vi "Excel_Quit.vi"(0 "Excel._Application in":refnum<k7>, 5 "Excel._Workbook in":refnum<k7>, 7 "save changes?":bool, 11 "error in":errorcluster, 12 "Close Application":bool, 13 "Close Report":bool) -> (4 "Excel._Application out":refnum<k7>, 6 "Excel._Workbook out":refnum<k7>, 15 "error out":errorcluster)   [LabVIEW 2020, in "NI_ReportGenerationToolkit.lvlib"]
uses:
  <vilib>/addons/_office/NI_ReportGenerationToolkit.lvlib
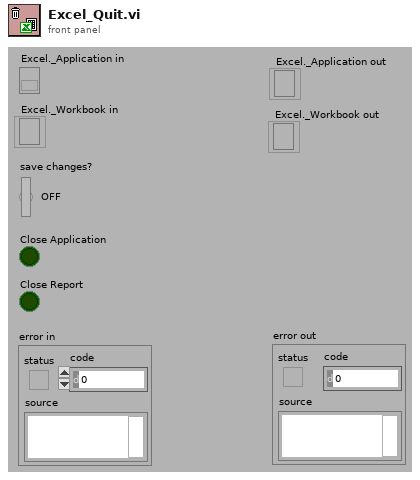
[diagram p1: front panel]
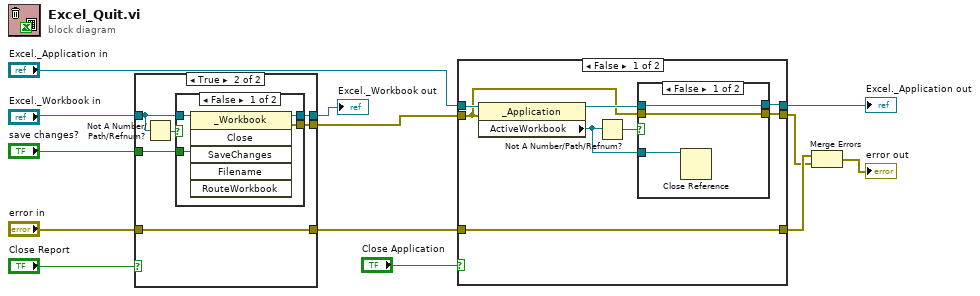
[diagram p0: block diagram]
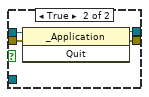
[diagram p2: hidden frame]
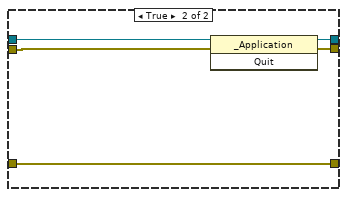
[diagram p3: hidden frame]
diagram:
  n1 = case shown="True" "Close Report" {
    tunnel: "save changes?" -> [_ w21]
    tunnel: [w14 w20] -> w4
    tunnel: "error in" -> [w14 w20]
    tunnel: "Excel._Workbook in" -> [w15 w17]
    tunnel: [w15 w19] -> w6
    tunnel: [_ w18] -> w3
    frame False {
    }
    frame True {
      n2 = Not A Number/Path/Refnum?(number/path/refnum=w17) -> (NaN/Path/Refnum?=w16:bool)
      n3 = case shown="False" w16 {
        tunnel: w21 -> [w25 _]
        tunnel: w17 -> [w24 w26]
        tunnel: [w23 w26] -> w19
        tunnel: [w22 _] -> w18
        frame False {
          n4 = invoke class="_Workbook" method="Close"(reference=w24, "SaveChanges"=w25) -> (reference out=w23:refnum<k7>, error out=w22:errorcluster)  [unwired: 4 in, 4 out]
        }
        frame True {
        }
      }
    }
  }
  "Excel._Workbook out" <- w6
  n5 = case shown="False" "Close Application" {
    tunnel: [w33 w46] -> w12
    tunnel: [w32 w45] -> w1
    tunnel: w4 -> [w34 w44]
    tunnel: [w34 w44] -> w2
    tunnel: "Excel._Application in" -> [w31 w43]
    tunnel: w3 -> [w28 w42]
    frame False {
      n6 = property class="_Application"(reference=w31, error in=w28) -> (reference out=w30:refnum<k7>, "ActiveWorkbook"=w27:refnum<k7>)  [unwired: 1 out]
      n7 = Not A Number/Path/Refnum?(number/path/refnum=w27) -> (NaN/Path/Refnum?=w29:bool)
      n8 = case shown="False" w29 {
        tunnel: [w37 w41] -> w33
        tunnel: [w36 w40] -> w32
        tunnel: w30 -> [w37 w39]
        tunnel: w28 -> [w36 w38]
        tunnel: w27 -> [w35 _]
        frame False {
          n9 = Close Reference(reference=w35) -> ()  [unwired: 1 in, 1 out]
        }
        frame True {
          n10 = invoke class="_Application" method="Quit"(reference=w39, error in=w38) -> (reference out=w41:refnum<k7>, error out=w40:errorcluster)  [unwired: 1 in, 1 out]
        }
      }
    }
    frame True {
      n11 = invoke class="_Application" method="Quit"(reference=w43, error in=w42) -> (reference out=w46:refnum<k7>, error out=w45:errorcluster)  [unwired: 1 in, 1 out]
    }
  }
  "Excel._Application out" <- w12
  n12 = Merge Errors(w2, w1) -> (→"error out":errorcluster)
